vi "Interrogate_register.vi"(6 "Address override":i32, 8 "error in (no error)":errorcluster, 9 "UUT Index":i32, 10 "Register mutli-protocol location":T2={"General Parameter name"="", "MODBUS Register"=0, "Profibus"={"Friendly name"="", "PA"={"Slot"=0, "Index"=0}, "DP"={"Slot"=0, "Index"=0}, "Tag"=""}, "Fieldbus"={"Parameter name"="", "Fieldbus Block"="", "Fieldbus Tag"=""}, "data type"=enum."float", "DeviceNET"={"ClassId"=102, "InstanceId"=1, "AttributeId"=12}, "Cluster"={"address"=0, "Mode"=0}, "Length"=0} {"Cluster"."Mode" items=["None", "MODBUS", "HART", "Profibus DP", "Profibus PA", "Fieldbus", "DeviceNET"]}, 11 "MODBUS in":refnum<class "USB_MODBUS.lvclass">) -> (0 "error out":errorcluster, 1 "Parameter name":string, 2 "output":sgl, 3 "MODBUS out":refnum<class "USB_MODBUS.lvclass">, 4 "output cluster":T1)   [LabVIEW 2016, in "USB_MODBUS.lvclass"]
uses:
  USB_MODBUS.lvclass
  Typedef/comm_variable_definition.ctl
  Typedef/Comm_mode_and_address_type.ctl
  Typedef/Comm_mode_type_combo.ctl
  USB_MODBUS.lvclass/USB_MODBUS.ctl
  Protocol Class/Protocol.lvclass
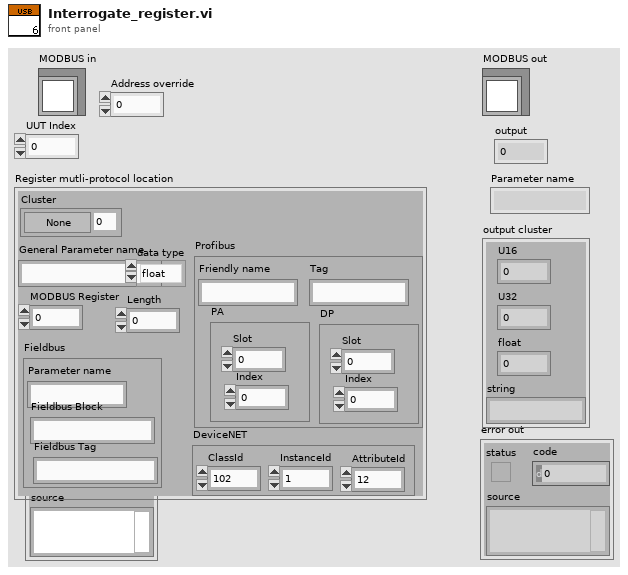
[diagram p1: front panel]
types:
  T1 = cluster{"U16":u16, "U32":u32, "float":sgl, "string":string}
  T2 = typedef "comm_variable_definition.ctl" = cluster{"General Parameter name":string, "MODBUS Register":i32, "Profibus":cluster{"Friendly name":string, "PA":cluster{"Slot":i32, "Index":i32}, "DP":cluster{"Slot":i32, "Index":i32}, "Tag":string}, "Fieldbus":cluster{"Parameter name":string, "Fieldbus Block":string, "Fieldbus Tag":string}, "data type":enum16{"float", "UINT", "UINT32", "STRING"}, "DeviceNET":cluster{"ClassId":u16, "InstanceId":u16, "AttributeId":u8}, "Cluster":T3, "Length":i32}
  T3 = typedef "Comm_mode_and_address_type.ctl" = cluster{"address":i32, "Mode":T4}
  T4 = typedef "Comm_mode_type_combo.ctl" = u16
  T5 = typedef "MODBUS parameters type.ctl" = cluster{"Mode":enum16{"RTU", "ASCII"}, "Default Slave Address":u8, "MODBUS timeout":u32, "Baud Rate":u32, "Parity":u16, "Flow Control":u16}
  T6 = cluster{"Device address":i32, "Switch index":i32}[]
  T7 = cluster{"Device address":i32, "Switch index":i32}
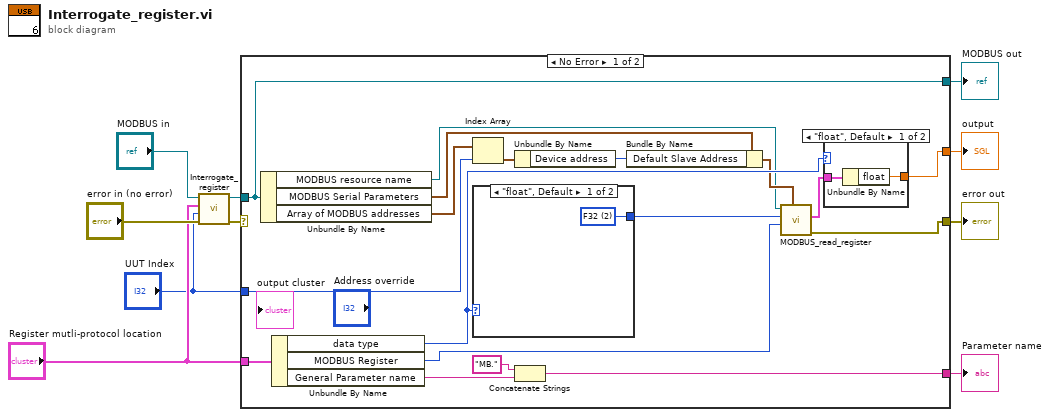
[diagram p0: block diagram]
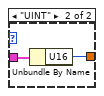
[diagram p2: hidden frame]
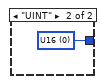
[diagram p3: hidden frame]
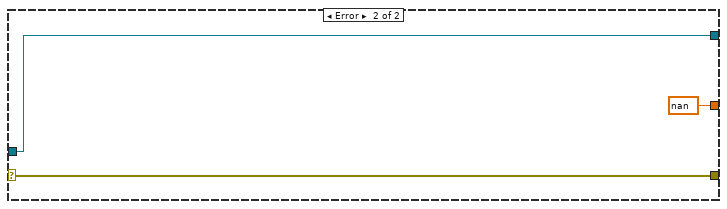
[diagram p4: hidden frame]
diagram:
  n1 = call-parent "Interrogate_register.vi"("error in (no error)"="error in (no error)", "UUT Index"="UUT Index", "Register mutli-protocol location"="Register mutli-protocol location", "Protocol in"="MODBUS in") -> ("error out"=w8:errorcluster, "Protocol out"=w7:refnum<class "USB_MODBUS.lvclass">)  [unwired: 3 in, 3 out]
  n2 = case shown="No Error" w8 {
    selector: w8 -> [_ w37]
    tunnel: "Register mutli-protocol location" -> [w28 _]
    tunnel: [w27 sgl nan ("type single")] -> w2
    tunnel: [w26 w37] -> w3
    tunnel: "UUT Index" -> [w16 _]
    tunnel: w7 -> [w18 w35]
    tunnel: [w18 w35] -> w4
    tunnel: [w11 _] -> w1
    frame No Error {
      n3 = Unbundle By Name(w18) -> ("MODBUS resource name"=w19:refnum<visa-resource-name>, "MODBUS Serial Parameters"=w21:T5, "Array of MODBUS addresses"=w17:T6)
      n4 = Unbundle By Name(w28) -> ("data type"=w23:enum16{"float", "UINT", "UINT32", "STRING"}, "MODBUS Register"=w25:i32, "General Parameter name"=w12:string)
      n5 = Index Array(array=w17, index=w16) -> (element=w15:T7)
      n6 = case shown="\"float\", Default" w23 {
        tunnel: [w33 w34] -> w24
        frame "float", Default {
          w33 = u16 2 items=["U16", "U32", "F32", "A8", "A12", "A16", "A22"] ("data type")
        }
        frame "UINT" {
          w34 = u16 0 items=["U16", "U32", "F32", "A8", "A12", "A16", "A22"] ("data type")
        }
      }
      n7 = Unbundle By Name(w15) -> ("Device address"=w14:i32)
      n8 = Concatenate Strings("MB." ("Protocol name"), w12) -> (w11:string)
      n9 = Bundle By Name(cluster=w21, "Default Slave Address"=w14) -> (w20:T5)
      n10 = call "MODBUS_read_register.vi"("MODBUS Serial Parameters"=w20, "Register"=w25, "Length"=w24, "VISA resource name"=w19) -> ("error out"=w26:errorcluster, "output cluster"=w22:T1)  [unwired: 4 in, 2 out]
      n11 = case shown="\"float\", Default" w23 {
        tunnel: [w29 w31] -> w27
        tunnel: w22 -> [w30 w32]
        frame "float", Default {
          n12 = Unbundle By Name(w30) -> ("float"=w29:sgl)
        }
        frame "UINT" {
          n13 = Unbundle By Name(w32) -> ("U16"=w31:u16)
        }
      }
    }
    frame Error {
    }
  }
  "error out" <- w3
  "MODBUS out" <- w4
  "output" <- w2
  "Parameter name" <- w1
